vi "Core UI Configuraton Extractor API.vi"(8 "error constant":errorcluster, 11 "General Config DVR In":refnum<data-value>) -> (0 "error out":errorcluster, 3 "Module Template Config":T1)   [LabVIEW 2021, in "Core UI.lvlib"]
doc: "This method extracts is a Poliphormic method used to read each module configuration."
uses:
  Core UI.lvlib
  Typedefs/Application Configuration.ctl
  Module Template/Typedefs/Config.ctl
  Typedefs/Config.ctl
  Configuration/Configuration.lvlib
  Module Template/Module Template.lvlib
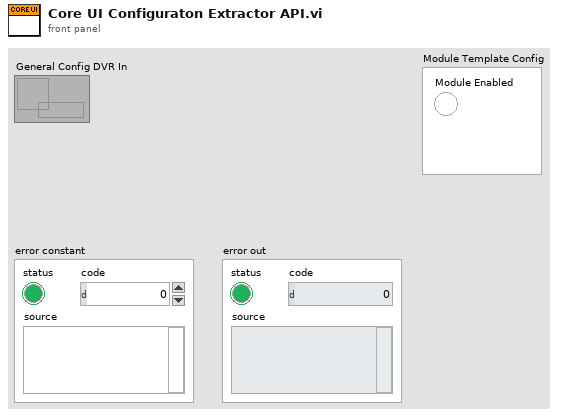
[diagram p1: front panel]
types:
  T1 = typedef "Core UI.lvlib/Config.ctl" = cluster{"Module Enabled":bool}
  T2 = typedef "Configuration.lvlib/Application Configuration.ctl" = cluster{"Module Template Config":T3, "Core UI Config":T1}
  T3 = typedef "Module Template.lvlib/Config.ctl" = cluster{"Module Enabled":bool}
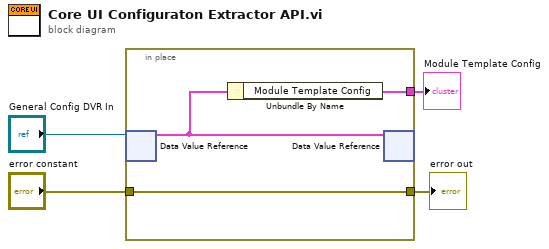
[diagram p0: block diagram]
diagram:
  n1 = in-place {
    in-place-border: [w5] -> w1
    in-place-border: "error constant" -> [w6]
    in-place-border: [w6] -> w2
    n2 = in-place-dvr #1("General Config DVR In") -> (w7:T2)  [unwired: 1 out]
    n3 = Unbundle By Name(w7) -> ("Module Template Config"=w5:T3)
    n4 = in-place-dvr #1(w7) -> ()  [unwired: 2 out]
  }
  "error out" <- w2
  "Module Template Config" <- w1
